vi "UT1E3.vi"() -> ()   [LabVIEW 2025]
uses:
  Control 2.ctl
panel:
  in  "Boolean":bool
  out "Sh":bool
  out "A3":bool
  out "A2":bool
  out "A1":bool
  out "A0":bool
  out "Piezas Delgadas":dbl
  out "Piezas Gruesas":dbl
  in  "Encendido":bool
  in  "Apagado":bool
  out "Slide 3":T1 scale=0.0..120.0
  # "Delgado"
  # "Grueso"
  # "Pieza Gruesa"
  # "Pieza Delgada"
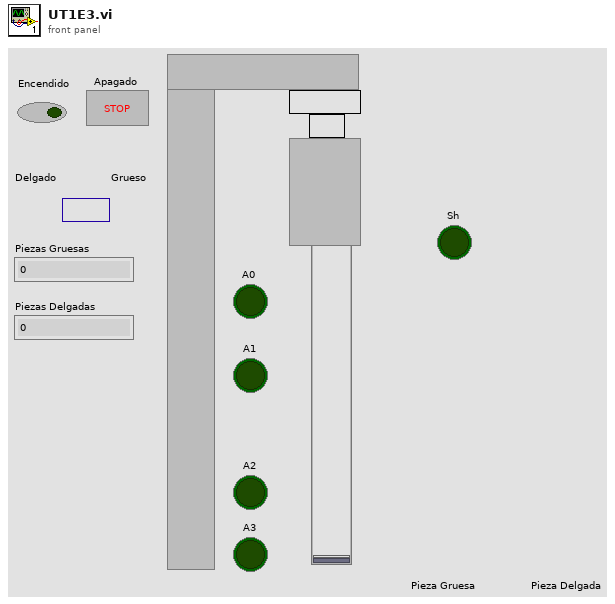
[diagram p1: front panel]
types:
  T1 = typedef "Control 2.ctl" = dbl
  T2 = enum16{"Inicio", "Seleccion", "PG1", "PG2", "PG3", "PD1"}
  T3 = enum16{"Inicio", "Seleccion", "PG1", "PG2", "PG3", "PD1", "PG5"}
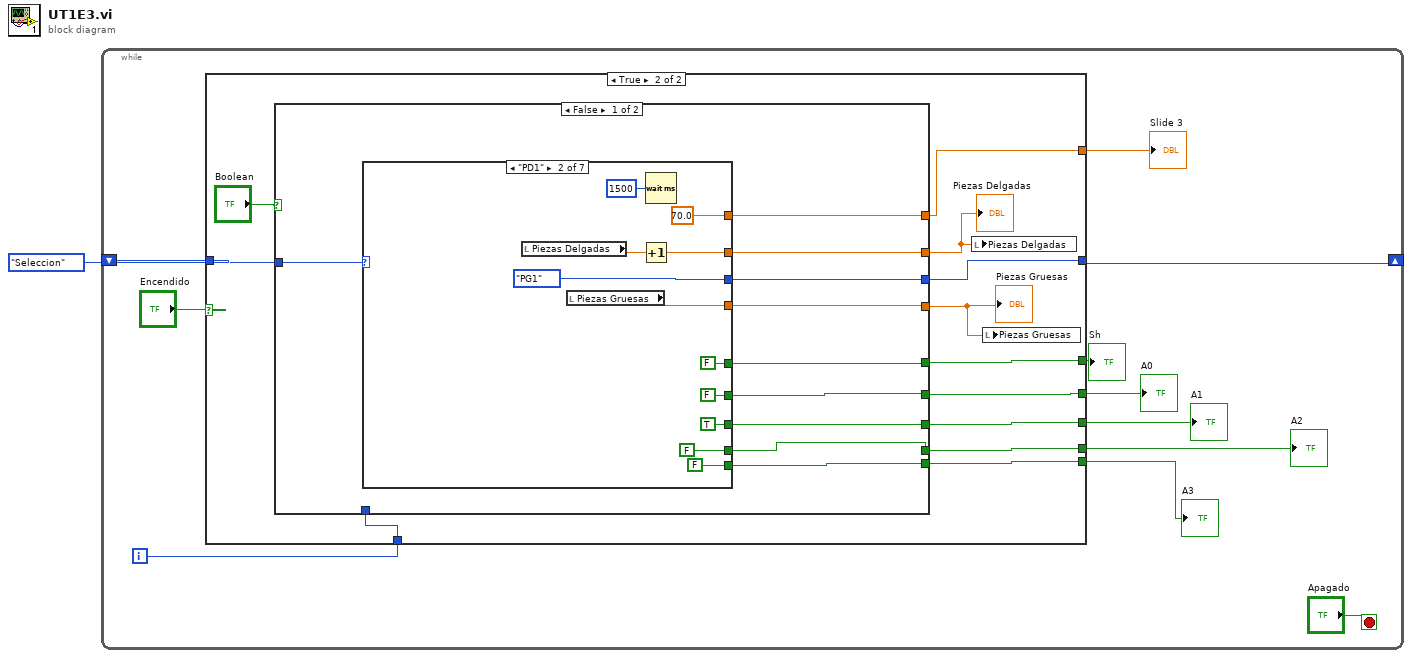
[diagram p0: block diagram]
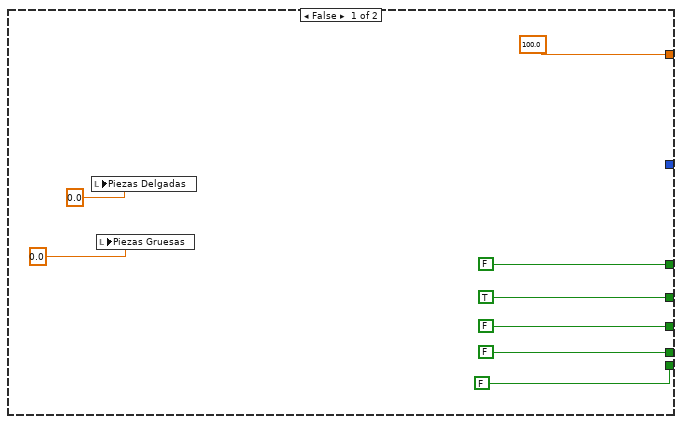
[diagram p2: hidden frame]
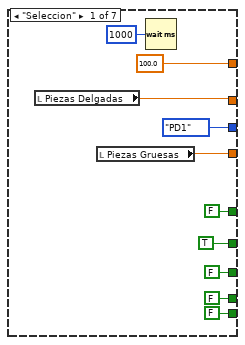
[diagram p3: hidden frame]
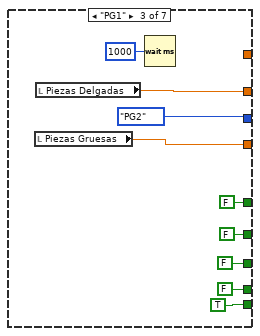
[diagram p4: hidden frame]
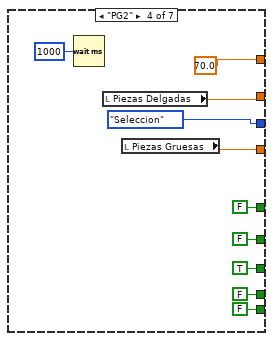
[diagram p5: hidden frame]
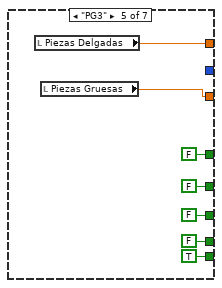
[diagram p6: hidden frame]
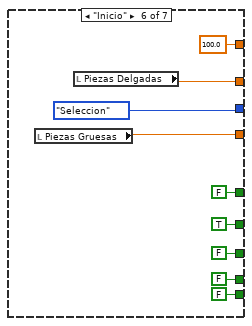
[diagram p7: hidden frame]
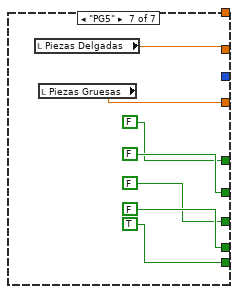
[diagram p8: hidden frame]
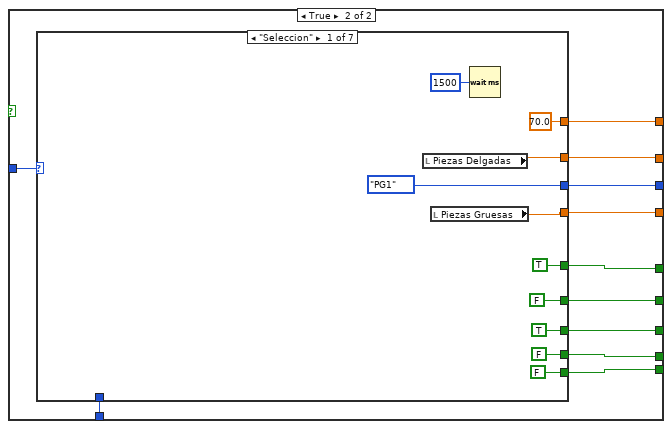
[diagram p9: hidden frame]
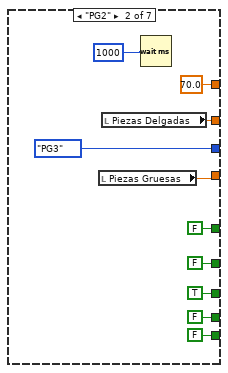
[diagram p10: hidden frame]
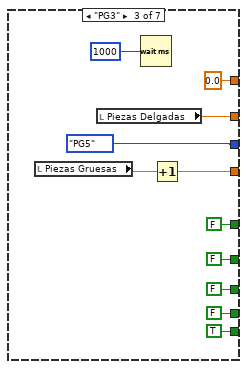
[diagram p11: hidden frame]
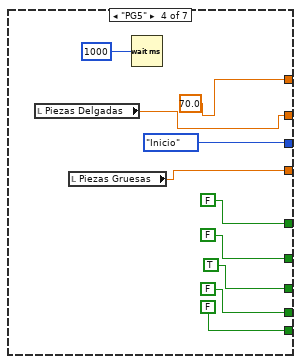
[diagram p12: hidden frame]
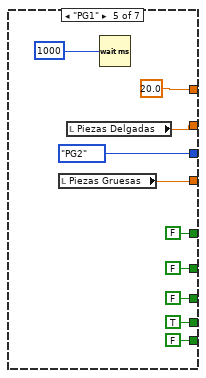
[diagram p13: hidden frame]
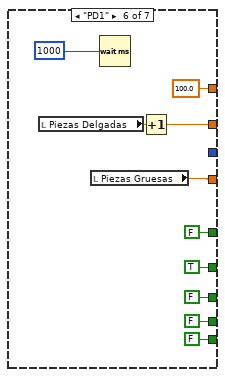
[diagram p14: hidden frame]
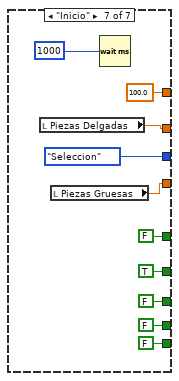
[diagram p15: hidden frame]
diagram:
  n1 = while {
    shift-right: [w10] -> _
    shift-left: T2."Seleccion" -> [w11]
    i -> [w8]
    stop <- "Apagado" stop-if-true
    n2 = case shown="True" "Encendido" {
      tunnel: w11 -> [_ w32]
      tunnel: [_ w31] -> w10
      tunnel: w8 -> [_ w30]
      tunnel: [FALSE ("Sh") w29] -> w7
      tunnel: [TRUE ("A0") w28] -> w6
      tunnel: [FALSE ("A1") w27] -> w5
      tunnel: [FALSE ("A2") w26] -> w4
      tunnel: [FALSE ("A3") w25] -> w3
      tunnel: [100.0 w21] -> w2
      frame False {
        n3 = local write "Piezas Delgadas"(0.0) -> ()
        n4 = local write "Piezas Gruesas"(0.0) -> ()
      }
      frame True {
        n5 = case shown="False" "Boolean" {
          tunnel: [w34 w115] -> w21
          tunnel: w32 -> [w42 w114]
          tunnel: [w33 w116] -> w31
          tunnel: w30 -> [_ w113]
          tunnel: [w36 w112] -> w24
          tunnel: [w35 w111] -> w23
          tunnel: [w37 w110] -> w29
          tunnel: [w38 w109] -> w28
          tunnel: [w39 w108] -> w27
          tunnel: [w40 w107] -> w26
          tunnel: [w41 w106] -> w25
          frame False {
            n6 = case shown="\"PD1\"" w42 {
              tunnel: [T2."PD1" T2."PG1" T2."PG2" T2."Seleccion" _ T2."Seleccion" _] -> w33
              tunnel: [100.0 ("Slide 3") 70.0 ("Slide 3") _ 70.0 _ 100.0 ("Slide 3") _] -> w34
              tunnel: [w49 w59 w72 w82 w89 w98 w100] -> w35
              tunnel: [TRUE ("A0") FALSE ("A0") FALSE ("A0") FALSE ("A0") FALSE ("A0") TRUE ("A0") FALSE ("A0")] -> w38
              tunnel: [FALSE ("A3") FALSE ("A3") TRUE ("A3") FALSE ("A3") TRUE ("A3") FALSE ("A3") TRUE ("A3")] -> w41
              tunnel: [FALSE ("A1") TRUE ("A1") FALSE ("A1") TRUE ("A1") FALSE ("A1") FALSE ("A1") FALSE ("A1")] -> w39
              tunnel: [FALSE ("A2") FALSE ("A2") FALSE ("A2") FALSE ("A2") FALSE ("A2") FALSE ("A2") FALSE ("A2")] -> w40
              tunnel: [FALSE ("Sh") FALSE ("Sh") FALSE ("Sh") FALSE ("Sh") FALSE ("Sh") FALSE ("Sh") FALSE ("Sh")] -> w37
              tunnel: [w43 w53 w66 w76 w83 w92 w99] -> w36
              frame "Seleccion" {
                n7 = local read "Piezas Delgadas"() -> (w49:dbl)
                n8 = local read "Piezas Gruesas"() -> (w43:dbl)
                n9 = Wait (ms)(milliseconds to wait=u32 1000) -> ()  [unwired: 1 out]
              }
              frame "PD1" {
                n10 = local read "Piezas Delgadas"() -> (w60:dbl)
                n11 = local read "Piezas Gruesas"() -> (w53:dbl)
                n12 = Increment(x=w60) -> (x+1=w59:dbl)
                n13 = Wait (ms)(milliseconds to wait=u32 1500) -> ()  [unwired: 1 out]
              }
              frame "PG1" {
                n14 = local read "Piezas Gruesas"() -> (w66:dbl)
                n15 = local read "Piezas Delgadas"() -> (w72:dbl)
                n16 = Wait (ms)(milliseconds to wait=u32 1000) -> ()  [unwired: 1 out]
              }
              frame "PG2" {
                n17 = Wait (ms)(milliseconds to wait=u32 1000) -> ()  [unwired: 1 out]
                n18 = local read "Piezas Delgadas"() -> (w82:dbl)
                n19 = local read "Piezas Gruesas"() -> (w76:dbl)
              }
              frame "PG3" {
                n20 = local read "Piezas Delgadas"() -> (w89:dbl)
                n21 = local read "Piezas Gruesas"() -> (w83:dbl)
              }
              frame "Inicio" {
                n22 = local read "Piezas Gruesas"() -> (w92:dbl)
                n23 = local read "Piezas Delgadas"() -> (w98:dbl)
              }
              frame "PG5" {
                n24 = local read "Piezas Delgadas"() -> (w100:dbl)
                n25 = local read "Piezas Gruesas"() -> (w99:dbl)
              }
            }
          }
          frame True {
            n26 = case shown="\"Seleccion\"" w114 {
              tunnel: [T2."PG1" T2."PG3" T3."PG5" T3."Inicio" T2."PG2" _ T2."Seleccion"] -> w116
              tunnel: [70.0 ("Slide 3") 70.0 ("Slide 3") 0.0 ("Slide 3") 70.0 20.0 ("Slide 3") 100.0 ("Slide 3") 100.0 ("Slide 3")] -> w115
              tunnel: w113 -> [_ _ _ _ _ _ _]
              tunnel: [w123 w133 w144 w149 w164 w177 w186] -> w112
              tunnel: [w122 w132 w142 w150 w163 w175 w185] -> w111
              tunnel: [TRUE ("Sh") FALSE ("Sh") FALSE ("Sh") FALSE ("Sh") FALSE ("Sh") FALSE ("Sh") FALSE ("Sh")] -> w110
              tunnel: [FALSE ("A0") FALSE ("A0") FALSE ("A0") FALSE ("A0") FALSE ("A0") TRUE ("A0") TRUE ("A0")] -> w109
              tunnel: [TRUE ("A1") TRUE ("A1") FALSE ("A1") TRUE ("A1") FALSE ("A1") FALSE ("A1") FALSE ("A1")] -> w108
              tunnel: [FALSE ("A2") FALSE ("A2") FALSE ("A2") FALSE ("A2") TRUE ("A2") FALSE ("A2") FALSE ("A2")] -> w107
              tunnel: [FALSE ("A3") FALSE ("A3") TRUE ("A3") FALSE ("A3") FALSE ("A3") FALSE ("A3") FALSE ("A3")] -> w106
              frame "Seleccion" {
                n27 = local read "Piezas Delgadas"() -> (w122:dbl)
                n28 = local read "Piezas Gruesas"() -> (w123:dbl)
                n29 = Wait (ms)(milliseconds to wait=u32 1500) -> ()  [unwired: 1 out]
              }
              frame "PG2" {
                n30 = local read "Piezas Gruesas"() -> (w133:dbl)
                n31 = local read "Piezas Delgadas"() -> (w132:dbl)
                n32 = Wait (ms)(milliseconds to wait=u32 1000) -> ()  [unwired: 1 out]
              }
              frame "PG3" {
                n33 = local read "Piezas Gruesas"() -> (w143:dbl)
                n34 = local read "Piezas Delgadas"() -> (w142:dbl)
                n35 = Wait (ms)(milliseconds to wait=u32 1000) -> ()  [unwired: 1 out]
                n36 = Increment(x=w143) -> (x+1=w144:dbl)
              }
              frame "PG5" {
                n37 = local read "Piezas Delgadas"() -> (w150:dbl)
                n38 = local read "Piezas Gruesas"() -> (w149:dbl)
                n39 = Wait (ms)(milliseconds to wait=u32 1000) -> ()  [unwired: 1 out]
              }
              frame "PG1" {
                n40 = local read "Piezas Gruesas"() -> (w164:dbl)
                n41 = local read "Piezas Delgadas"() -> (w163:dbl)
                n42 = Wait (ms)(milliseconds to wait=u32 1000) -> ()  [unwired: 1 out]
              }
              frame "PD1" {
                n43 = local read "Piezas Delgadas"() -> (w176:dbl)
                n44 = local read "Piezas Gruesas"() -> (w177:dbl)
                n45 = Wait (ms)(milliseconds to wait=u32 1000) -> ()  [unwired: 1 out]
                n46 = Increment(x=w176) -> (x+1=w175:dbl)
              }
              frame "Inicio" {
                n47 = local read "Piezas Delgadas"() -> (w185:dbl)
                n48 = local read "Piezas Gruesas"() -> (w186:dbl)
                n49 = Wait (ms)(milliseconds to wait=u32 1000) -> ()  [unwired: 1 out]
              }
            }
          }
        }
        "Piezas Gruesas" <- w24
        "Piezas Delgadas" <- w23
        n50 = local write "Piezas Delgadas"(w23) -> ()
        n51 = local write "Piezas Gruesas"(w24) -> ()
      }
    }
    "A1" <- w5
    "A2" <- w4
    "A3" <- w3
    "Sh" <- w7
    "A0" <- w6
    "Slide 3" <- w2
  }
